vi "Finish Create.vi"(4 "Actor Ref":refnum<vi>, 6 "Creator Attributes":refnum<class "Attributes.lvclass">, 7 "Alias":string, 9 "Queue of Self Attributes":refnum<queue>, 10 "Actor in":refnum<class "Actor.lvclass">) -> (0 "Error out":errorcluster, 1 "Teardown Create":bool, 2 "Actor out":refnum<class "Actor.lvclass">)   [LabVIEW 2020, in "jettl.lvlib" / "Actor.lvlib"]
uses:
  Actor.lvlib
  Actor/Actor.lvclass
  Attributes/Attributes/Attributes.lvclass
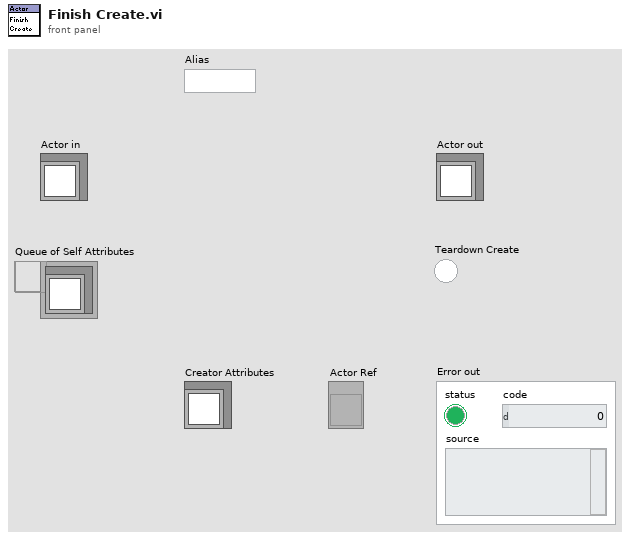
[diagram p1: front panel]
types:
  T1 = typedef "jettl.lvlib/Actor.lvlib/Msg Set.ctl" = set{refnum<class "Msg.lvclass">}
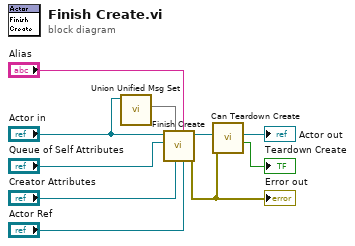
[diagram p0: block diagram]
diagram:
  n1 = call-dynamic "Union Unified Msg Set.vi"("Get Actor in"="Actor in") -> ("Unified Msg Set"=w10:T1)  [unwired: 10 in]
  n2 = call-dynamic "Finish Create.vi"("Actor Ref"="Actor Ref", "Alias"="Alias", "Creator Attributes"="Creator Attributes", "Unified Msg Set"=w10, "Queue of Self Attributes"="Queue of Self Attributes", "Actor in"="Actor in") -> ("Error out"=w4:errorcluster, "Actor out"=w3:refnum<class "Actor.lvclass">)  [unwired: 4 in]
  "Error out" <- w4
  n3 = call "Can Teardown Create.vi"("Error in"=w4, "Actor in"=w3) -> ("Teardown Create"=→"Teardown Create":bool, "Actor out"=→"Actor out":refnum<class "Actor.lvclass">)  [unwired: 8 in]
